vi "CliSetParam.vi"(0 "ref in":u64, 5 "ParamNumber":i32(ring)=3 items=["Local Port"=1, "Remote Port"=2, "Ping Timeout (ms)"=3, "Send Timeout (ms)"=4, "Recv Timeout (ms)"=5, "Work Interval (ms)"=6, "Source REF"=7, "Destination REF"=8, "Source TSAP"=9, "PDU Request"=10, "Max Clients"=11, "BSend Timeout (ms)"=12, "BRecv Timeout (ms)"=13, "Recovery Time (ms)"=14, "Keep Alive Time (ms)"=15], 7 "Param Value":i64, 11 "error in (no error)":errorcluster) -> (4 "ref out":u64, 6 "Result":i32, 15 "error out":errorcluster)   [LabVIEW 2020, in "Snap7.lvlib"]
uses:
  Snap7.lvlib
  windows/lv_snap7.dll
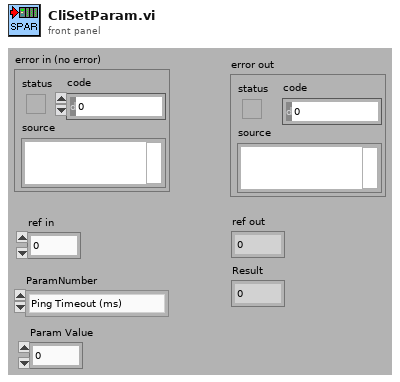
[diagram p1: front panel]
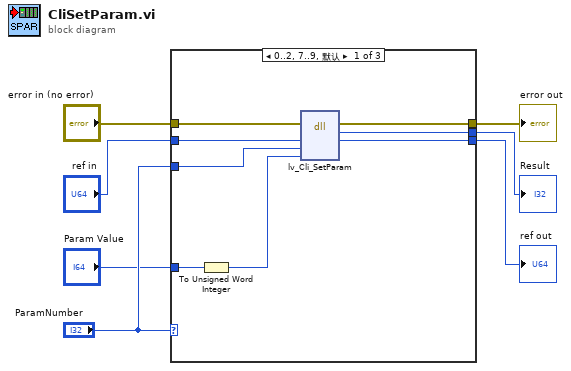
[diagram p0: block diagram]
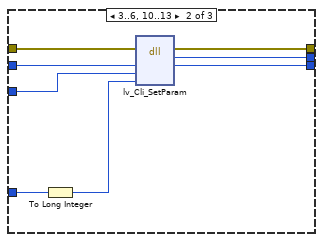
[diagram p2: hidden frame]
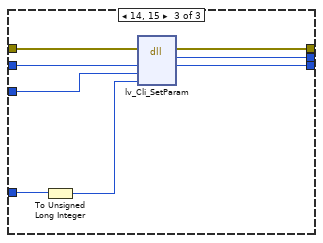
[diagram p3: hidden frame]
diagram:
  n1 = case shown="0..2, 7..9, 默认" "ParamNumber" {
    tunnel: "ref in" -> [w14 w23 w30]
    tunnel: [w11 w22 w27] -> w6
    tunnel: [w10 w21 w26] -> w5
    tunnel: "error in (no error)" -> [w15 w20 w31]
    tunnel: [w12 w19 w28] -> w3
    tunnel: "ParamNumber" -> [w13 w18 w29]
    tunnel: "Param Value" -> [w9 w16 w25]
    frame 0..2, 7..9, Default {
      n2 = To Unsigned Word Integer(number=w9) -> (unsigned 16bit integer=w8:u16)
      n3 = dll-call lib="PTH2fabs CUsersFeng项目HLCEPS300-2性能试验台SourcesSnap7libwindowslv_snap7.dll" fn="lv_Cli_SetParam"(error in=w15, "Client"=w14, "ParamNumber"=w13, "ParamValue"=w8) -> (error out=w12:errorcluster, "return type"=w11:i32, "Client"=w10:u64)  [unwired: 4 in, 1 out]
    }
    frame 3..6, 10..13 {
      n4 = To Long Integer(number=w16) -> (32bit integer=w17:i32)
      n5 = dll-call lib="PTH2fabs CUsersFeng项目HLCEPS300-2性能试验台SourcesSnap7libwindowslv_snap7.dll" fn="lv_Cli_SetParam"(error in=w20, "Client"=w23, "ParamNumber"=w18, "ParamValue"=w17) -> (error out=w19:errorcluster, "return type"=w22:i32, "Client"=w21:u64)  [unwired: 4 in, 1 out]
    }
    frame 14, 15 {
      n6 = To Unsigned Long Integer(number=w25) -> (unsigned 32bit integer=w24:u32)
      n7 = dll-call lib="PTH2fabs CUsersFeng项目HLCEPS300-2性能试验台SourcesSnap7libwindowslv_snap7.dll" fn="lv_Cli_SetParam"(error in=w31, "Client"=w30, "ParamNumber"=w29, "ParamValue"=w24) -> (error out=w28:errorcluster, "return type"=w27:i32, "Client"=w26:u64)  [unwired: 4 in, 1 out]
    }
  }
  "Result" <- w6
  "ref out" <- w5
  "error out" <- w3
